vi "Main.vi"() -> ()   [LabVIEW 2026]
doc: "This template is for the Queued Message Handler design pattern.\n\nThe Event Handling Loop generates messages based on user interface actions.\n\nThe Message Handling Loop processes messages generated by the Event Handling Loop, or by other messages. The messages are string values, so new messages can be added easily to the Message Cases case structure in the Message Handling Loop. Each message cluster can also provide an optional value for Message Data, which is a variant that can be converted to whatever message-specific data is required."
uses:
  SubVIs/Controls/PCO_Config.ctl
  SubVIs/Controls/UI Data.ctl
  <instrlib>/PCO_SDK/File Group 0/vi.lib/Excelitas PCO GmbH/pco.labview/camera/Camera.lvclass
  SubVIs/Controls/TypeDef_FGV.ctl
  <instrlib>/PCO_SDK/File Group 0/vi.lib/Excelitas PCO GmbH/pco.labview/camera/Controls/binning.ctl
  SubVIs/QMH/Message Queue/Enqueue Message (Single).vi
  SubVIs/QMH/Message Queue/Message Queue.lvlib
  SubVIs/QMH/User Event - Stop/User Event - Stop.lvlib
panel:
  in  "Image Index":u32 max=9
  in  "Saving path":path
  in  "# of frames":u16=1 min=1 step=1
  out "FFT":T1(plugin-control)
  out "Camera":T1(plugin-control)
  in  "Stop live":bool
  in  "FFT?":bool
  in  "Grab":bool
  in  "Live":bool
  in  "PCO_Config":T2={"Exposure time (s)"=0.1, "TriggerMode"=0, "ROI X0"=1, "ROI Y0"=1, "ROI X1"=2048, "ROI Y1"=2048, "Binning"=1} {"TriggerMode" items=["auto sequence", "software trigger", "external exposure start", "external exposure control"]}
  out "Image dimensions (px)":dbl[](array[numeric])=[2048.0, 2048.0]
  out "Current task":string="\"Exit\" button pressed"
  in  "Exit":bool
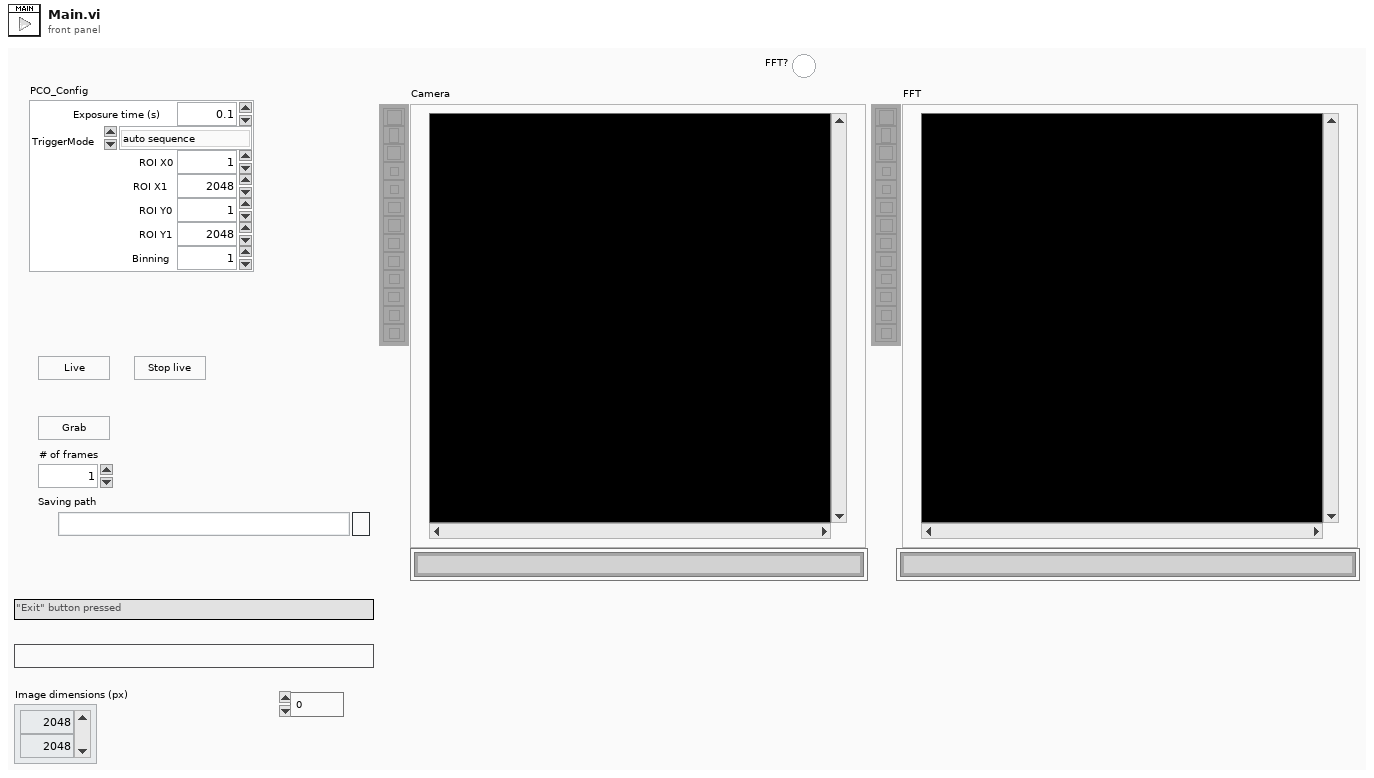
[diagram p1: front panel]
types:
  T1 = typedef "IMAQ Image.ctl" = refnum<image>
  T2 = typedef "PCO_Config.ctl" = cluster{"Exposure time (s)":dbl, "TriggerMode":u16, "ROI X0":u16, "ROI Y0":u16, "ROI X1":u16, "ROI Y1":u16, "Binning":u8}
  T3 = typedef "UI Data.ctl" = cluster{"Data Display Ref":refnum<vi>, "Exit Button Ref":refnum<vi>, "Message":string}
  T4 = typedef "Message Queue.lvlib/All Message Queues.ctl" = cluster{"UI":refnum<queue>, "Camera loop":refnum<queue>, "Display loop":refnum<queue>}
  T5 = typedef "TypeDef_FGV.ctl" = enum16{"Initialize", "Write", "Read"}
  T6 = typedef "Camera.lvclass/binning.ctl" = cluster{"vert":u16, "horz":u16, "mode":u16}
  T7 = cluster{"exposure_time_s":dbl, "delay_time_s":dbl, "roi":cluster{"x0":u64, "y0":u64, "x1":u64, "y1":u64}, "timestamp_mode":u16, "pixelrate":u32, "trigger_mode":u16, "acquire_mode":u16, "metadata_mode":u16, "noisefilter_mode":u16, "pixel_format":u32, "binning":T6, "auto_exposure":cluster{"region":u16, "min_exposure_s":dbl, "max_exposure_s":dbl}}
  T8 = enum16{"sequence", "sequence non blocking", "ring buffer", "fifo", "sequence_dpcore", "sequence_non_blocking_dpcore", "ring_buffer_dpcore", "fifo_dpcore", "tif", "multitif", "pcoraw", "b16", "dicom", "multidicom", "camram_ring", "camram_segment"}
  T9 = enum16{"Undefined", "Mono8", "Mono16", "BGRA8", "RGBA8", "BGRA16", "RGBA16", "CompressedMono8"}
  T10 = typedef "Image Type" = u32
  T11 = cluster{"serial":u32, "type":u16, "sub_type":u16, "interface_type":u16, "bit_resolution":u16, "min_exposure_time_s":dbl, "max_exposure_time_s":dbl, "min_exposure_step_s":dbl, "min_delay_time_s":dbl, "max_delay_time_s":dbl, "min_delay_step_s":dbl, "min_width":u64, "min_height":u64, "max_width":u64, "max_height":u64, "roi_step_horz":u64, "roi_step_vert":u64, "roi_symmetric_horz":bool, "roi_symmetric_vert":bool, "has_timestamp_mode":bool, "has_timestamp_mode_ascii_only":bool, "pixelrate_vec":u32[], "has_acquire_mode":bool, "has_ext_acquire_mode":bool, "has_metadata_mode":bool, "has_ram":bool, "binning_horz_vec":u16[], "binning_vert_vec":u16[], "has_average_binning":bool, "pixel_format_vec":u32[], "has_trigger_mode_extexpctrl":bool}
  T12 = cluster{"dwImgCounter":u32, "lvTimestamp":timestamp, "dwMicroSeconds":u32}[]
  T13 = cluster{"Plane 4 (alpha)":u16, "Plane 1 (Red)":u16, "Plane 2 (Green)":u16, "Plane 3 (Blue)":u16}[][][]
  T14 = cluster{"dwImgCounter":u32, "lvTimestamp":timestamp, "dwMicroSeconds":u32}
  T15 = typedef "IMAQ AVI2 Refnum.ctl" = refnum<k20>
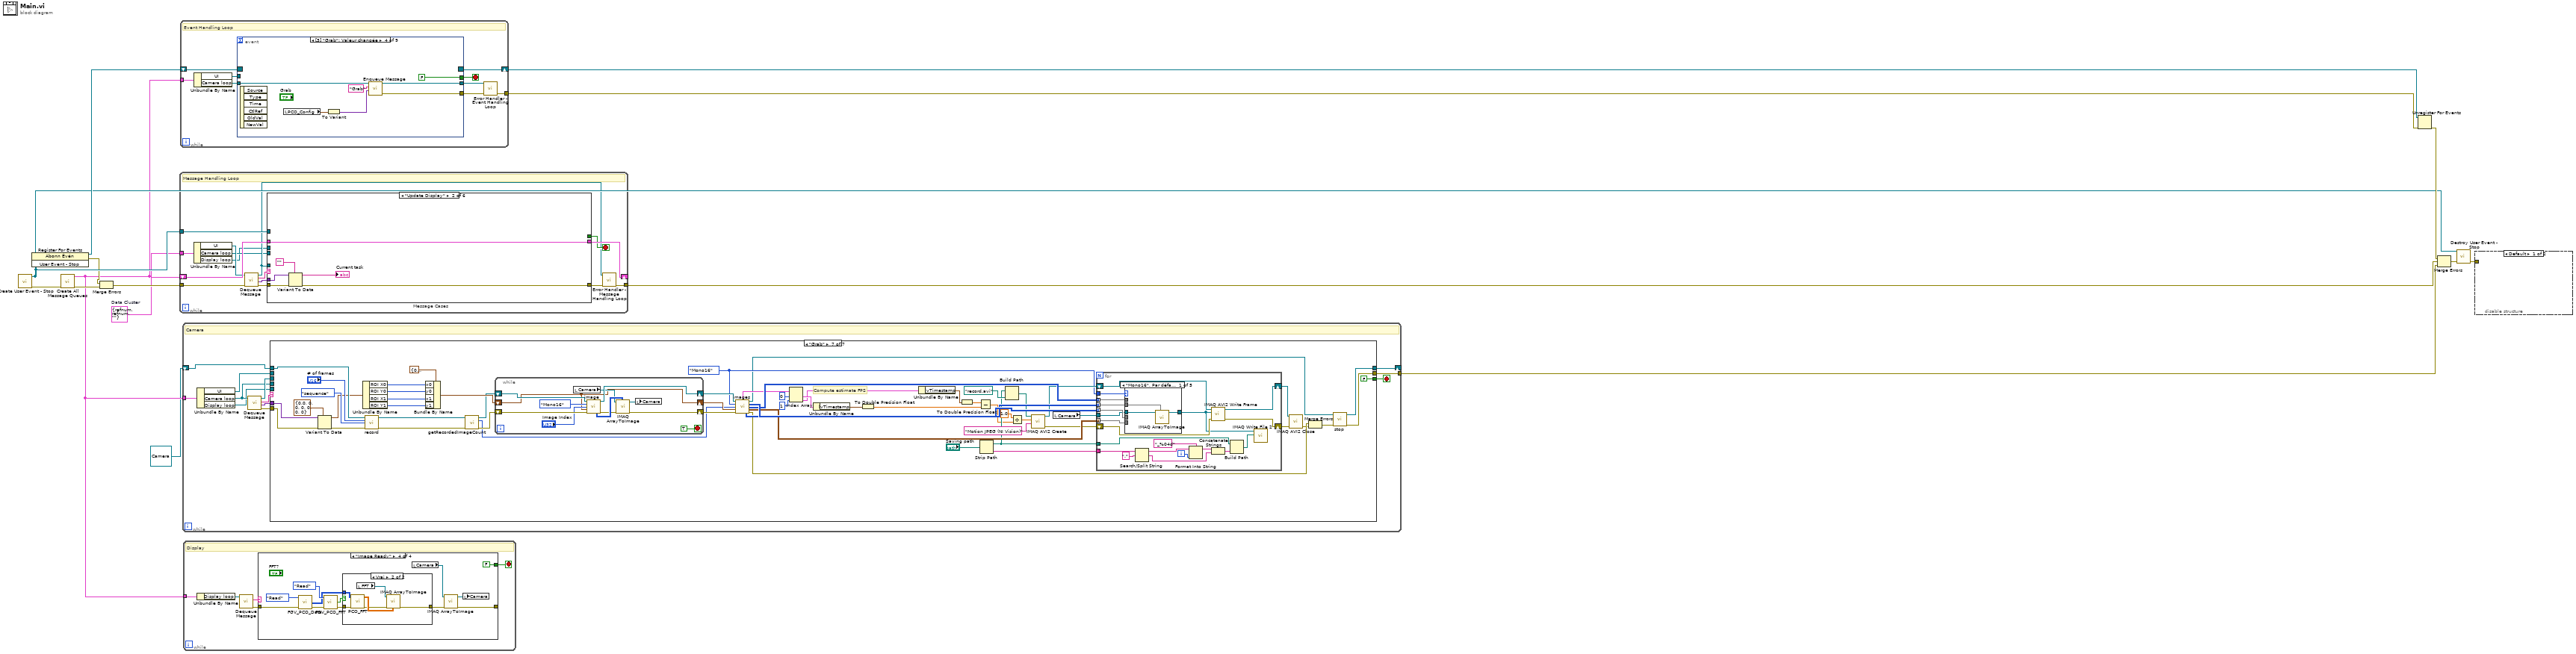
[diagram p0: block diagram]
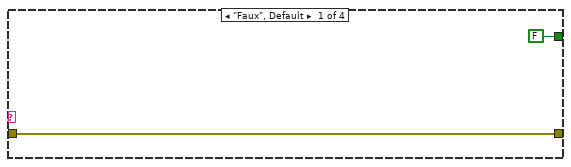
[diagram p2: hidden frame]
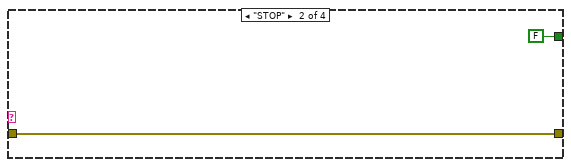
[diagram p3: hidden frame]
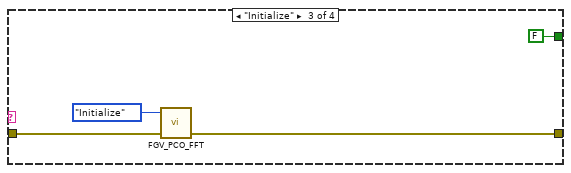
[diagram p4: hidden frame]
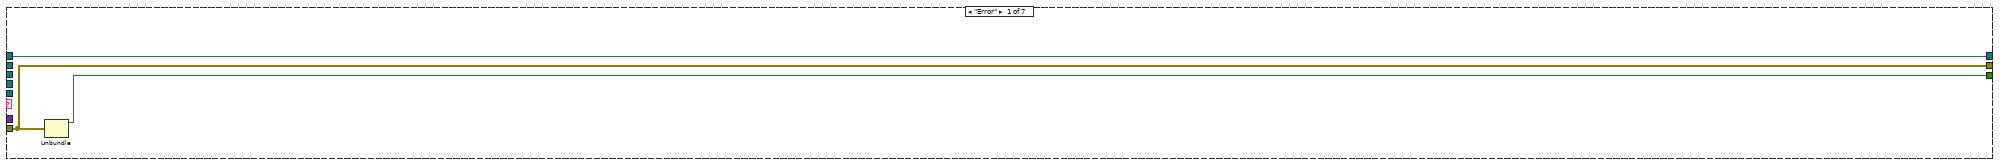
[diagram p6: hidden frame]
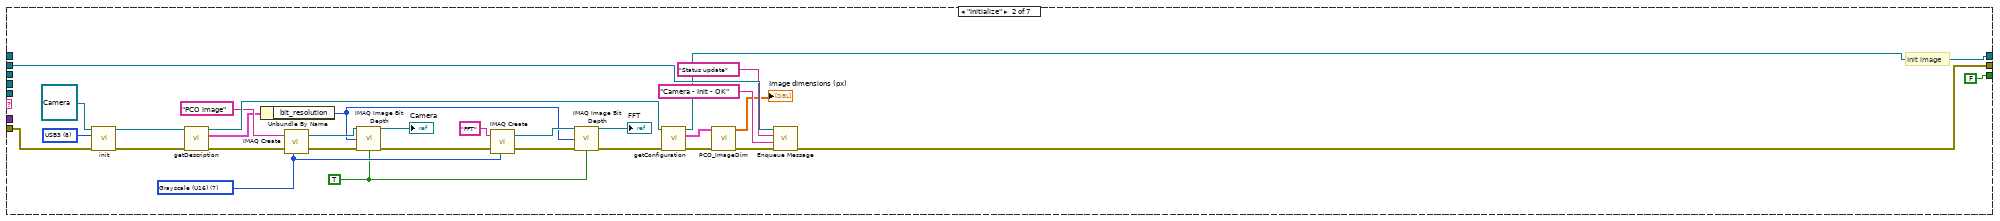
[diagram p7: hidden frame]
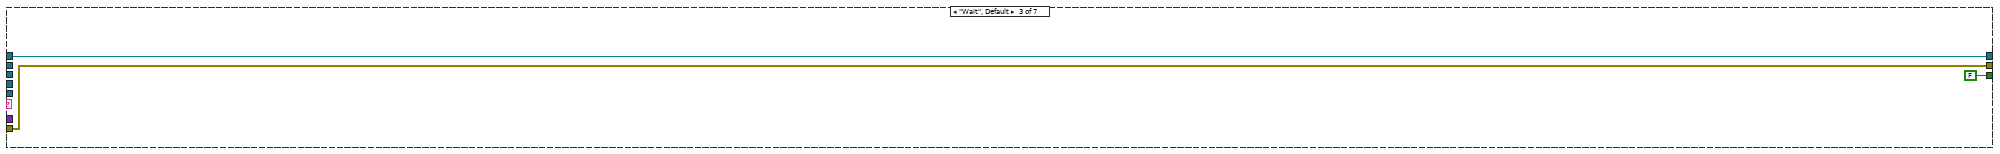
[diagram p8: hidden frame]
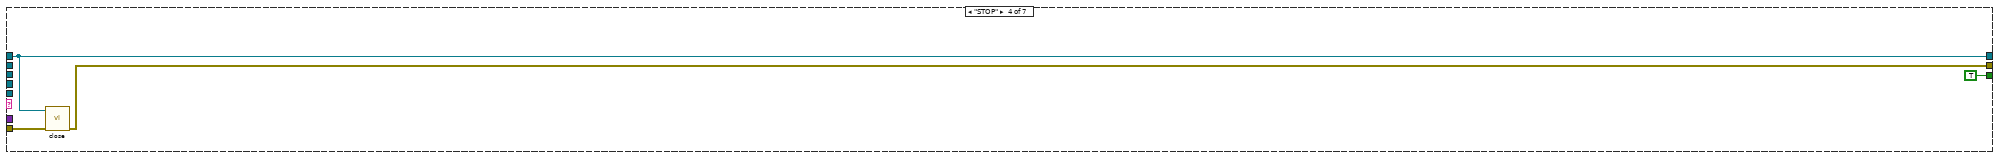
[diagram p9: hidden frame]
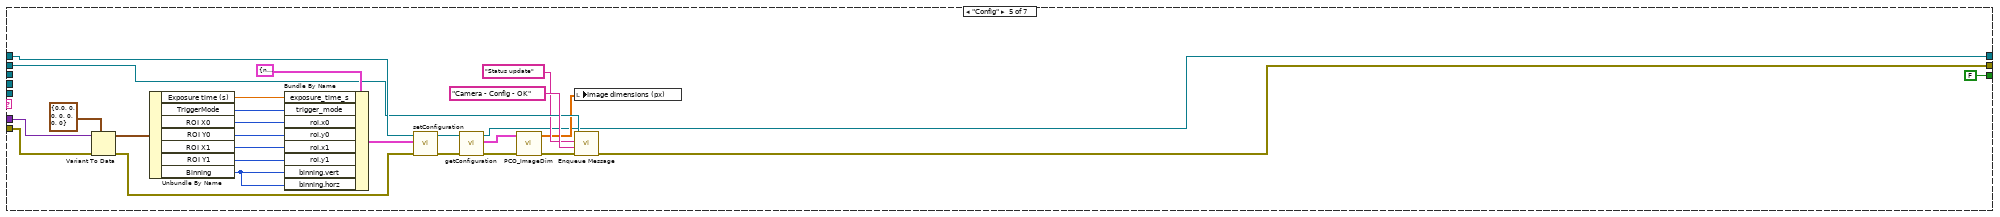
[diagram p10: hidden frame]
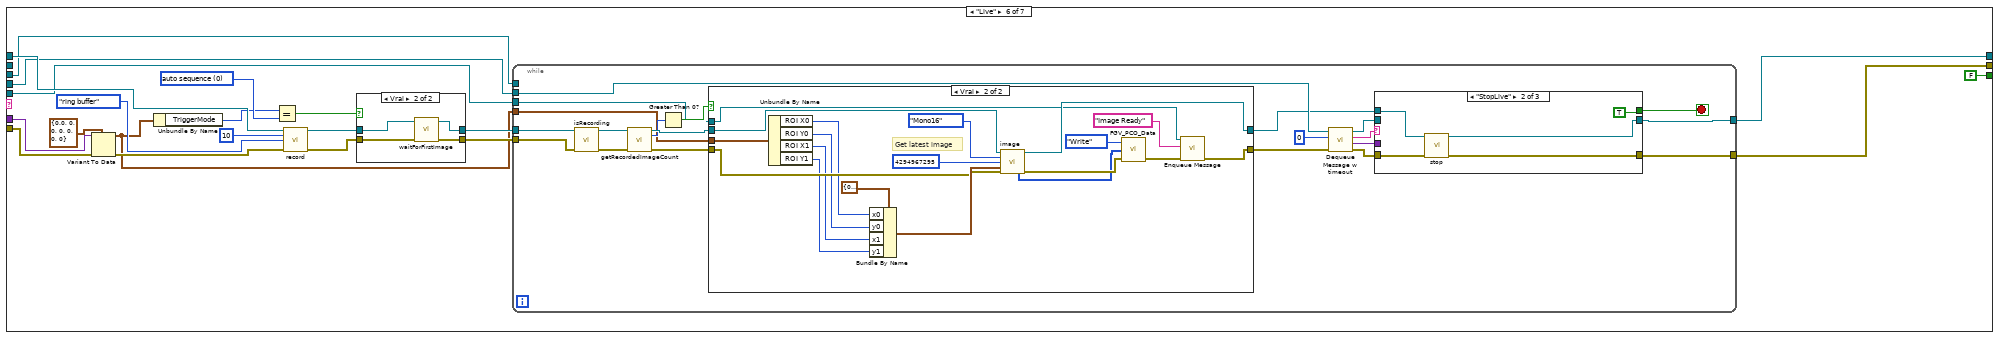
[diagram p11: hidden frame]
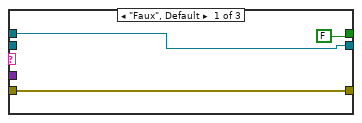
[diagram p12: hidden frame]
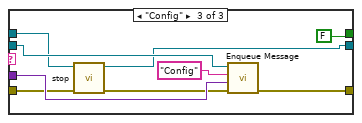
[diagram p13: hidden frame]
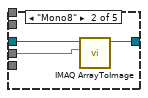
[diagram p16: hidden frame]
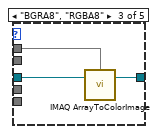
[diagram p17: hidden frame]
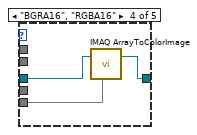
[diagram p18: hidden frame]
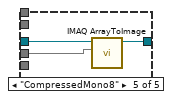
[diagram p19: hidden frame]
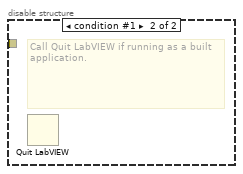
[diagram p20: hidden frame]
diagram:
  w4 = T3 {"Data Display Ref"=refnum, "Exit Button Ref"=refnum, "Message"=""}  # Data Cluster
  n1 = call "Create User Event - Stop.vi"() -> ("error out"=w14:errorcluster, "User Event - Stop"=w7:refnum<user-event>)  [unwired: 10 in]
  n2 = register-events(w7) -> (reference out=w8:refnum<event-registration>, error out=w5:errorcluster)  [unwired: 2 in]
  n3 = call "Create All Message Queues.vi"("error in (no error)"=w14) -> ("error out"=w16:errorcluster, "Message Queues out"=w2:T4)  [unwired: 9 in]
  n4 = Merge Errors(w5, w16) -> (w6:errorcluster)
  n5 = while {
    shift-right: [w30] -> _
    shift-left: w4 -> [w31]
    tunnel: w7 -> [w28]
    tunnel: w6 -> [w27]
    tunnel: [w22] -> w15
    tunnel: w2 -> [w20]
    stop <- w29 stop-if-true
    # "Message Handling Loop"
    n6 = Unbundle By Name(w20) -> ("UI"=w19:refnum<queue>, "Camera loop"=w18:refnum<queue>, "Display loop"=w17:refnum<queue>)
    n7 = call "Dequeue Message.vi"("error in (no error)"=w27, "Message Queue"=w19) -> ("error out"=w26:errorcluster, "Message Data"=w24:variant, "Message"=w25:string, "dup Message Queue"=w23:refnum<queue>)  [unwired: 6 in]
    n8 = case "Message Cases" shown="\"Update Display\"" w25 {
      tunnel: w23 -> [w34 _ _ w56 w70 _]
      tunnel: w26 -> [w39 w45 w52 w58 w71 w79]
      tunnel: [w40 w42 w47 w53 w66 w79] -> w21
      tunnel: w31 -> [w38 w46 w51 w57 w78 w80]
      tunnel: [w37 w46 w51 w57 w78 w80] -> w30
      tunnel: [_ _ _ _ TRUE _] -> w29
      tunnel: w24 -> [_ w44 w50 _ w74 _]
      tunnel: w28 -> [_ _ _ _ w76 _]
      tunnel: w18 -> [_ _ _ _ w69 _]
      tunnel: w17 -> [_ _ _ _ w59 _]
      frame "Initialize" {
        w32 = "Initial Message" ("Initial Message")
        n9 = control-ref of="Current task"() -> (w33:refnum<vi>)
        n10 = control-ref of="Exit"() -> (w36:refnum<vi>)
        n11 = Bundle By Name(cluster=w38, "Data Display Ref"=w33, "Exit Button Ref"=w36, "Message"=w32) -> (w37:T3)
        n12 = call-poly "Enqueue Message.vi"("error in (no error)"=w39, "Message Data"=w32, "Message"="Update Display", "Message Queue"=w34) -> ("error out"=w40:errorcluster)  [unwired: 6 in, 1 out]
      }
      frame "Update Display" {
        n13 = Variant To Data(error in=w45, type="", Variant=w44) -> (data=→"Current task":string, error out=w42:errorcluster)
      }
      frame "Error" {
        n14 = Variant To Data(error in=w52, type=errorcluster {"status"=FALSE, "code"=0, "source"=""} ("error constant"), Variant=w50) -> (data=w48:errorcluster, error out=w47:errorcluster)
        n15 = call <vilib>:"Simple Error Handler.vi"("error in (no error)"=w48) -> ()  [unwired: 4 in, 5 out]
      }
      frame "Confirm Quit" {
        n16 = call-poly "Enqueue Message.vi"("Priority Message? (F)"=TRUE, "error in (no error)"=w58, "Message"="Exit", "Message Queue"=w56) -> ("error out"=w53:errorcluster)  [unwired: 6 in, 1 out]
      }
      frame "Exit" {
        n17 = Variant To Data(error in=w71, type=errorcluster {"status"=FALSE, "code"=0, "source"=""} ("error constant"), Variant=w74) -> (error out=w67:errorcluster)  [unwired: 1 out]
        n18 = Release Queue(queue=w70, error in (no error)=w67) -> (error out=w65:errorcluster)  [unwired: 1 in, 2 out]
        n19 = call-poly "Enqueue Message.vi"("error in (no error)"=w65, "Message"="STOP", "Message Queue"=w69) -> ("error out"=w73:errorcluster, "dup Message Queue"=w72:refnum<queue>)  [unwired: 7 in]
        n20 = Release Queue(queue=w72, error in (no error)=w73) -> (error out=w61:errorcluster)  [unwired: 1 in, 2 out]
        n21 = call-poly "Enqueue Message.vi"("error in (no error)"=w61, "Message"="STOP", "Message Queue"=w59) -> ("error out"=w62:errorcluster, "dup Message Queue"=w63:refnum<queue>)  [unwired: 7 in]
        n22 = Release Queue(queue=w63, error in (no error)=w62) -> (error out=w60:errorcluster)  [unwired: 1 in, 2 out]
        n23 = call "Fire User Event - Stop.vi"("error in (no error)"=w60, "User Event - Stop"=w76) -> ("error out"=w66:errorcluster)  [unwired: 9 in]
      }
      frame Default {
      }
    }
    n24 = call "Error Handler - Message Handling Loop.vi"("error in (no error)"=w21, "Message Queue"=w23) -> ("dup error in"=w22:errorcluster)  [unwired: 8 in, 1 out]
  }
  n25 = while {
    shift-right: [w88] -> w11
    shift-left: w8 -> [w89]
    tunnel: [w84] -> w9
    tunnel: w2 -> [w81]
    stop <- w86 stop-if-true
    # "Event Handling Loop"
    n26 = Unbundle By Name(w81) -> ("UI"=w83:refnum<queue>, "Camera loop"=w82:refnum<queue>)
    n27 = event shown="[3] \"Grab\": Valeur changée" {
      selector: w89 -> [_ _ _ _ _ _ _ _ _]
      dyn-events: [_ _ _ _ _ _ _ _ _] -> w88
      timeout: _ -> [_ _ _ _ _ _ _ _ _]
      tunnel: [FALSE ("Discard?") FALSE ("Discard?") _ FALSE ("Discard?") FALSE ("Discard?") FALSE ("Discard?") FALSE ("Discard?") FALSE ("Discard?") TRUE ("Discard?")] -> w86
      tunnel: w83 -> [w95 w105 _ _ w123 _ w131 w138 w142]
      tunnel: [w94 w101 w108 w115 w121 w126 errorcluster {"status"=FALSE, "code"=0, "source"=""} ("error out") w132 errorcluster {"status"=FALSE, "code"=0, "source"=""} ("error out")] -> w87
      tunnel: [w93 w105 w107 w116 w123 w125 w131 w137 w142] -> w85
      tunnel: w82 -> [_ w99 w106 w117 _ w127 _ _ _]
      event Panel Close? {
        n28 = event-data() -> ()  [unwired: 1 in, 1 out]
        n29 = call-poly "Enqueue Message.vi"("Priority Message? (F)"=TRUE, "Message"="Confirm Quit", "Message Queue"=w95) -> ("error out"=w94:errorcluster, "dup Message Queue"=w93:refnum<queue>)  [unwired: 7 in]
        n30 = event-data("Discard?"=TRUE) -> ()  [unwired: 1 in, 1 out]
      }
      event Value Change {
        n31 = event-data() -> ()  [unwired: 1 in, 6 out]
        n32 = To Variant(anything="PCO_Config") -> (Variant=w102:variant)
        n33 = Flush Queue(queue=w99) -> (queue out=w97:refnum<queue>, error out=w98:errorcluster)  [unwired: 1 in, 1 out]
        n34 = call-poly "Enqueue Message.vi"("error in (no error)"=w98, "Message Data"=w102, "Message"="Config", "Message Queue"=w97) -> ("error out"=w101:errorcluster)  [unwired: 6 in, 1 out]
      }
      event "Live": Value Change {
        n35 = event-data() -> ()  [unwired: 1 in, 6 out]
        n36 = local read "PCO_Config"() -> (w111:T2)
        n37 = To Variant(anything=w111) -> (Variant=w110:variant)
        n38 = call-poly "Enqueue Message.vi"("Message Data"=w110, "Message"="Live", "Message Queue"=w106) -> ("error out"=w108:errorcluster, "dup Message Queue"=w107:refnum<queue>)  [unwired: 7 in]
      }
      event "Grab": Value Change {
        n39 = event-data() -> ()  [unwired: 1 in, 6 out]
        n40 = local read "PCO_Config"() -> (w113:T2)
        n41 = To Variant(anything=w113) -> (Variant=w112:variant)
        n42 = call-poly "Enqueue Message.vi"("Message Data"=w112, "Message"="Grab", "Message Queue"=w117) -> ("error out"=w115:errorcluster, "dup Message Queue"=w116:refnum<queue>)  [unwired: 7 in]
      }
      event "FFT?": Value Change {
        n43 = event-data() -> ("NewVal"=w119:bool)  [unwired: 1 in]
        n44 = call "FGV_PCO_FFT.vi"("FFT?"=w119, "Action"=TypeDef_FGV."Write") -> ("error out"=w121:errorcluster)  [unwired: 2 in, 1 out]
      }
      event "Stop live": Value Change {
        n45 = event-data() -> ()  [unwired: 1 in, 6 out]
        n46 = call-poly "Enqueue Message.vi"("Message"="StopLive", "Message Queue"=w127) -> ("error out"=w126:errorcluster, "dup Message Queue"=w125:refnum<queue>)  [unwired: 8 in]
      }
      event Application Instance Close {
        n47 = event-data() -> ()  [unwired: 1 in, 1 out]
      }
      event "Exit": Value Change {
        n48 = event-data() -> ()  [unwired: 1 in, 1 out]
        n49 = call-poly "Enqueue Message.vi"("Priority Message? (F)"=TRUE, "Message Data"=errorcluster {"status"=FALSE, "code"=0, "source"=""} ("error constant"), "Message"="Exit", "Message Queue"=w138) -> ("error out"=w132:errorcluster, "dup Message Queue"=w137:refnum<queue>)  [unwired: 6 in]
      }
      event User Event {
        n50 = event-data() -> ()  [unwired: 1 in, 1 out]
        n51 = local write "Current task"("\"Exit\" button pressed" ("VI Stopped")) -> ()
      }
    }
    n52 = call "Error Handler - Event Handling Loop.vi"("error in (no error)"=w87, "Message Queue"=w85) -> ("dup error in"=w84:errorcluster)  [unwired: 8 in, 1 out]
  }
  n53 = while {
    tunnel: [w150] -> w3
    tunnel: w2 -> [w148]
    shift-right: [w146] -> _
    shift-left: refnum<class "Camera.lvclass"> refnum ("Camera out") -> [w145]
    stop <- w151 stop-if-true
    # "Camera"
    n54 = Unbundle By Name(w148) -> ("UI"=w147:refnum<queue>, "Camera loop"=w144:refnum<queue>, "Display loop"=w143:refnum<queue>)
    n55 = call "Dequeue Message.vi"("Message Queue"=w144) -> ("error out"=w154:errorcluster, "Message Data"=w152:variant, "Message"=w153:string, "dup Message Queue"=w149:refnum<queue>)  [unwired: 7 in]
    n56 = case shown="\"Grab\"" w153 {
      tunnel: w154 -> [w157 w181 w191 w194 w221 w238 w357]
      tunnel: w152 -> [_ _ _ _ w220 w234 w356]
      tunnel: w147 -> [_ w188 _ _ w205 _ _]
      tunnel: [w156 FALSE ("status") FALSE ("status") TRUE FALSE ("status") FALSE ("status") FALSE ("status")] -> w151
      tunnel: [w157 w173 w191 w193 w204 w226 w311] -> w150
      tunnel: w149 -> [_ _ _ _ _ w229 _]
      tunnel: [w155 w178 w190 w192 w196 w225 w309] -> w146
      tunnel: w145 -> [w155 _ w190 w192 w215 w242 w363]
      tunnel: w144 -> [_ _ _ _ _ w228 _]
      tunnel: w143 -> [_ _ _ _ _ w227 _]
      frame "Error" {
        n57 = Unbundle(w157) -> ("status"=w156:bool)  [unwired: 2 out]
      }
      frame "Initialize" {
        w159 = TRUE ("Get/Set Bit Depth? (Set)")
        w164 = T10 7 items=["Grayscale (U8)", "Grayscale (I16)", "Grayscale (SGL)", "Complex (CSG)", "RGB (U32)", "HSL (U32)", "RGB (U64)", "Grayscale (U16)"] ("Image Type")
        w180 = u16 8 items=["FireWire"=1, "GenICam"=3, "GigE"=5, "USB"=6, "CameraLinkME4"=7, "USB3"=8, "CLHS"=11, "All"=65535] ("interface")
        # "Init image"
        n58 = call-dynamic "init.vi"("Camera in"=refnum<class "Camera.lvclass"> refnum, "interface"=w180, "error in (no error)"=w181) -> ("Camera out"=w184:refnum<class "Camera.lvclass">, "error out"=w183:errorcluster)  [unwired: 6 in]
        n59 = call-dynamic "getDescription.vi"("error in (no error)"=w183, "Camera in"=w184) -> ("error out"=w167:errorcluster, "description"=w170:T11, "Camera out"=w179:refnum<class "Camera.lvclass">)  [unwired: 7 in]
        n60 = Unbundle By Name(w170) -> ("bit_resolution"=w160:u16)
        n61 = call "IMAQ Create"("Image Name"="PCO Image", "Image Type"=w164, "error in (no error)"=w167) -> ("New Image"=w169:T1, "error out"=w168:errorcluster)  [unwired: 2 in]
        n62 = call "IMAQ Image Bit Depth"("Image"=w169, "Bit Depth (0)"=w160, "error in (no error)"=w168, "Get/Set Bit Depth? (Set)"=w159) -> ("Image Out"=→"Camera":T1, "error out"=w165:errorcluster)  [unwired: 9 in, 1 out]
        n63 = call "IMAQ Create"("Image Name"="FFT", "Image Type"=w164, "error in (no error)"=w165) -> ("New Image"=w162:T1, "error out"=w163:errorcluster)  [unwired: 2 in]
        n64 = call "IMAQ Image Bit Depth"("Image"=w162, "Bit Depth (0)"=w160, "error in (no error)"=w163, "Get/Set Bit Depth? (Set)"=w159) -> ("Image Out"=→"FFT":T1, "error out"=w158:errorcluster)  [unwired: 9 in, 1 out]
        n65 = call-dynamic "getConfiguration.vi"("error in (no error)"=w158, "Camera in"=w179) -> ("error out"=w176:errorcluster, "configuration"=w177:T7, "Camera out"=w178:refnum<class "Camera.lvclass">)  [unwired: 7 in]
        n66 = call "PCO_ImageDim.vi"("error in"=w176, "configuration"=w177) -> ("error out"=w175:errorcluster, "Dimensions"=→"Image dimensions (px)":dbl[])  [unwired: 8 in]
        n67 = call-poly "Enqueue Message.vi"("error in (no error)"=w175, "Message Data"="Camera - Init - OK", "Message"="Status update", "Message Queue"=w188) -> ("error out"=w173:errorcluster)  [unwired: 6 in, 1 out]
      }
      frame "Wait", Default {
      }
      frame "STOP" {
        n68 = call-dynamic "close.vi"("error in (no error)"=w194, "Camera in"=w192) -> ("error out"=w193:errorcluster)  [unwired: 9 in]
      }
      frame "Config" {
        n69 = Variant To Data(error in=w221, type=T2 {"Exposure time (s)"=0.0, "TriggerMode"=0, "ROI X0"=0, "ROI Y0"=0, "ROI X1"=0, "ROI Y1"=0, "Binning"=0} ("PCO_Config"), Variant=w220) -> (data=w217:T2, error out=w216:errorcluster)
        n70 = Unbundle By Name(w217) -> ("Exposure time (s)"=w213:dbl, "TriggerMode"=w212:u16, "ROI X0"=w207:u16, "ROI Y0"=w208:u16, "ROI X1"=w209:u16, "ROI Y1"=w210:u16, "Binning"=w211:u8)
        n71 = Bundle By Name(cluster=T7 {"exposure_time_s"=nan, "delay_time_s"=nan, "roi"={"x0"=18446744073709551615, "y0"=18446744073709551615, "x1"=18446744073709551615, "y1"=18446744073709551615}, "timestamp_mode"=65535, "pixelrate"=4294967295, "trigger_mode"=65535, "acquire_mode"=65535, "metadata_mode"=65535, "noisefilter_mode"=65535, "pixel_format"=4294967295, "binning"={"vert"=65535, "horz"=65535, "mode"=0}, "auto_exposure"={"region"=0, "min_exposure_s"=0.001, "max_exposure_s"=0.1}} ("configuration"), "exposure_time_s"=w213, "trigger_mode"=w212, "roi.x0"=w207, "roi.y0"=w208, "roi.x1"=w209, "roi.y1"=w210, "binning.vert"=w211, "binning.horz"=w211) -> (w214:T7)
        n72 = call-dynamic "setConfiguration.vi"("error in (no error)"=w216, "configuration"=w214, "Camera in"=w215) -> ("error out"=w198:errorcluster, "Camera out"=w199:refnum<class "Camera.lvclass">)  [unwired: 7 in]
        n73 = call-dynamic "getConfiguration.vi"("error in (no error)"=w198, "Camera in"=w199) -> ("error out"=w202:errorcluster, "configuration"=w201:T7, "Camera out"=w196:refnum<class "Camera.lvclass">)  [unwired: 7 in]
        n74 = call "PCO_ImageDim.vi"("error in"=w202, "configuration"=w201) -> ("error out"=w197:errorcluster, "Dimensions"=w200:dbl[])  [unwired: 8 in]
        n75 = local write "Image dimensions (px)"(w200) -> ()
        n76 = call-poly "Enqueue Message.vi"("error in (no error)"=w197, "Message Data"="Camera - Config - OK", "Message"="Status update", "Message Queue"=w205) -> ("error out"=w204:errorcluster)  [unwired: 6 in, 1 out]
      }
      frame "Live" {
        w236 = u16 0 items=["auto sequence", "software trigger", "external exposure start", "external exposure control"] ("TriggerMode")
        n77 = Variant To Data(error in=w238, type=T2 {"Exposure time (s)"=0.0, "TriggerMode"=0, "ROI X0"=0, "ROI Y0"=0, "ROI X1"=0, "ROI Y1"=0, "Binning"=0} ("PCO_Config"), Variant=w234) -> (data=w230:T2, error out=w237:errorcluster)
        n78 = Unbundle By Name(w230) -> ("TriggerMode"=w235:u16)
        n79 = Equal?(x=w235, y=w236) -> (x = y?=w233:bool)
        n80 = call-dynamic "record.vi"("Camera in"=w242, "num_images"=u32 10 ("dwImgCount"), "record_mode"=T8."ring buffer", "error in (no error)"=w237) -> ("Camera out"=w223:refnum<class "Camera.lvclass">, "error out"=w224:errorcluster)  [unwired: 10 in]
        n81 = case shown="Vrai" w233 {
          tunnel: w224 -> [w303 w308]
          tunnel: w223 -> [w304 w307]
          tunnel: [w304 w306] -> w231
          tunnel: [w303 w305] -> w232
          frame False {
          }
          frame True {
            n82 = call-dynamic "waitForFirstImage.vi"("error in (no error)"=w308, "Camera in"=w307) -> ("error out"=w305:errorcluster, "Camera out"=w306:refnum<class "Camera.lvclass">)  [unwired: 8 in]
          }
        }
        n83 = while {
          tunnel: w232 -> [w258]
          tunnel: w231 -> [w257]
          tunnel: w230 -> [w256]
          tunnel: w229 -> [_]
          tunnel: w228 -> [w254]
          tunnel: w227 -> [w252]
          tunnel: [w247] -> w226
          tunnel: [w246] -> w225
          stop <- w245 stop-if-true
          n84 = call-dynamic "isRecording.vi"("Camera in"=w257, "error in (no error)"=w258) -> ("Camera out"=w264:refnum<class "Camera.lvclass">, "error out"=w263:errorcluster)  [unwired: 11 in, 1 out]
          n85 = call-dynamic "getRecordedImageCount.vi"("Camera in"=w264, "error in (no error)"=w263) -> ("Camera out"=w261:refnum<class "Camera.lvclass">, "recorded_image_count"=w259:u32, "error out"=w262:errorcluster)  [unwired: 11 in]
          n86 = Greater Than 0?(x=w259) -> (x > 0?=w260:bool)
          n87 = case shown="Vrai" w260 {
            tunnel: [w282 w288] -> w255
            tunnel: w262 -> [w282 w299]
            tunnel: w261 -> [w283 w298]
            tunnel: [w283 w297] -> w248
            tunnel: w256 -> [_ w296]
            tunnel: w252 -> [_ w290]
            frame False {
            }
            frame True {
              # "Get latest image"
              n88 = Unbundle By Name(w296) -> ("ROI X0"=w295:u16, "ROI Y0"=w294:u16, "ROI X1"=w293:u16, "ROI Y1"=w292:u16)
              n89 = Bundle By Name(cluster=cluster{"x0":u64, "y0":u64, "x1":u64, "y1":u64} {"x0"=0, "y0"=0, "x1"=0, "y1"=0} ("roi"), "x0"=w295, "y0"=w294, "x1"=w293, "y1"=w292) -> (w300:cluster{"x0":u64, "y0":u64, "x1":u64, "y1":u64})
              n90 = call-dynamic "image.vi"("Camera in"=w298, "data_format"=T9."Mono16", "image_index"=u32 4294967295 ("dwImgIdx"), "roi"=w300, "error in (no error)"=w299) -> ("Camera out"=w297:refnum<class "Camera.lvclass">, "raw_image (U16)"=w284:u16[][], "error out"=w286:errorcluster)  [unwired: 2 in, 6 out]
              n91 = call "FGV_PCO_Data.vi"("error in"=w286, "Data"=w284, "Action"=TypeDef_FGV."Write") -> ("error out"=w285:errorcluster)  [unwired: 1 in, 1 out]
              n92 = call-poly "Enqueue Message.vi"("error in (no error)"=w285, "Message"="Image Ready", "Message Queue"=w290) -> ("error out"=w288:errorcluster)  [unwired: 7 in, 1 out]
            }
          }
          n93 = call "Dequeue Message w timeout.vi"("entrée d'erreur (pas d'erreur)"=w255, "timeout en ms (-1)"=0, "Message Queue"=w254) -> ("sortie d'erreur"=w250:errorcluster, "Message Data"=w249:variant, "Message"=w253:string, "Message Queue"=w251:refnum<queue>)  [unwired: 5 in]
          n94 = case shown="\"StopLive\"" w253 {
            tunnel: w251 -> [_ _ w281]
            tunnel: w250 -> [w266 w271 w276]
            tunnel: w249 -> [_ _ w279]
            tunnel: w248 -> [w267 w272 w277]
            tunnel: [w266 w270 w274] -> w247
            tunnel: [w267 w269 w278] -> w246
            tunnel: [FALSE TRUE FALSE] -> w245
            frame "Faux", Default {
            }
            frame "StopLive" {
              n95 = call-dynamic "stop.vi"("error in (no error)"=w271, "Camera in"=w272) -> ("error out"=w270:errorcluster, "Camera out"=w269:refnum<class "Camera.lvclass">)  [unwired: 8 in]
            }
            frame "Config" {
              n96 = call-dynamic "stop.vi"("error in (no error)"=w276, "Camera in"=w277) -> ("error out"=w275:errorcluster, "Camera out"=w278:refnum<class "Camera.lvclass">)  [unwired: 8 in]
              n97 = call-poly "Enqueue Message.vi"("error in (no error)"=w275, "Message Data"=w279, "Message"="Config", "Message Queue"=w281) -> ("error out"=w274:errorcluster)  [unwired: 6 in, 1 out]
            }
          }
        }
      }
      frame "Grab" {
        w315 = T9."Mono16" ("data_format")
        # "Compute estimate FPS"
        n98 = Variant To Data(error in=w357, type=T2 {"Exposure time (s)"=0.0, "TriggerMode"=0, "ROI X0"=0, "ROI Y0"=0, "ROI X1"=0, "ROI Y1"=0, "Binning"=0} ("PCO_Config"), Variant=w356) -> (data=w354:T2, error out=w355:errorcluster)
        n99 = Unbundle By Name(w354) -> ("ROI X0"=w353:u16, "ROI Y0"=w352:u16, "ROI X1"=w351:u16, "ROI Y1"=w350:u16)
        n100 = call-dynamic "record.vi"("Camera in"=w363, "num_images"="# of frames", "record_mode"=T8."sequence", "error in (no error)"=w355) -> ("Camera out"=w362:refnum<class "Camera.lvclass">, "error out"=w361:errorcluster)  [unwired: 10 in]
        n101 = Bundle By Name(cluster=cluster{"x0":u64, "y0":u64, "x1":u64, "y1":u64} {"x0"=0, "y0"=0, "x1"=0, "y1"=0} ("roi"), "x0"=w353, "y0"=w352, "x1"=w351, "y1"=w350) -> (w359:cluster{"x0":u64, "y0":u64, "x1":u64, "y1":u64})
        n102 = call-dynamic "getRecordedImageCount.vi"("Camera in"=w362, "error in (no error)"=w361) -> ("Camera out"=w348:refnum<class "Camera.lvclass">, "recorded_image_count"=w316:u32, "error out"=w349:errorcluster)  [unwired: 11 in]
        n103 = while {
          shift-right: [w411] -> w346
          shift-left: w348 -> [w413]
          shift-right: [w404] -> w347
          shift-left: w349 -> [w412]
          shift-right: [w403] -> w317
          shift-left: w359 -> [w403]
          stop <- TRUE stop-if-true
          n104 = local read "Camera"() -> (w408:T1)
          n105 = call-dynamic "image.vi"("Camera in"=w413, "data_format"=T9."Mono16", "image_index"="Image Index", "roi"=w403, "error in (no error)"=w412) -> ("Camera out"=w411:refnum<class "Camera.lvclass">, "raw_image (U16)"=w409:u16[][], "error out"=w405:errorcluster)  [unwired: 2 in, 6 out]
          n106 = call "IMAQ ArrayToImage"("Image Pixels (U16)"=w409, "error in (no error)"=w405, "Image"=w408) -> ("error out"=w404:errorcluster, "Image Out"=w407:T1)  [unwired: 7 in]
          n107 = local write "Camera"(w407) -> ()
        }
        n108 = call-dynamic "images.vi"("Camera in"=w346, "data_format"=w315, "image_count"=w316, "roi"=w317, "error in (no error)"=w347) -> ("timestamp_list"=w330:T12, "Camera out"=w310:refnum<class "Camera.lvclass">, "image_list (U8)"=w345:u8[][][], "image_list (U32)"=w343:u32[][][], "image_list (U64)"=w342:T13, "raw_image_list (U16)"=w344:u16[][][], "error out"=w337:errorcluster)  [unwired: 2 in, 2 out]
        n109 = Index Array(array=w330, index #1=0 ("index"), index #2=1 ("index")) -> (element #1=w327:T14, element #2=w326:T14)
        n110 = Unbundle By Name(w327) -> ("lvTimestamp"=w325:timestamp)
        n111 = To Double Precision Float(number=w325) -> (double precision float=w322:dbl)
        n112 = Unbundle By Name(w326) -> ("lvTimestamp"=w324:timestamp)
        n113 = To Double Precision Float(number=w324) -> (double precision float=w323:dbl)
        n114 = Subtract(x=w323, y=w322) -> (x-y=w321:dbl)
        n115 = Strip Path(path="Saving path") -> (stripped path=w331:path, name=w334:string)
        n116 = Build Path(base path=w331, name or relative path=path "record.avi") -> (appended path=w332:path)
        n117 = Divide(x=1.0, y=w321) -> (x/y=w319:dbl)
        n118 = call "IMAQ AVI2 Create"("Codec"="Motion JPEG (NI Vision)", "Frames Per Second"=w319, "AVI Path"=w332) -> ("error out"=w341:errorcluster, "AVI Refnum"=w340:T15)  [unwired: 7 in]
        n119 = local read "Camera"() -> (w335:T1)
        n120 = for {
          tunnel: w345 -> [w386] mode=indexing
          tunnel: w344 -> [w385] mode=indexing
          tunnel: w343 -> [w384] mode=indexing
          tunnel: w342 -> [w383] mode=indexing
          shift-right: [w379] -> w338
          shift-left: w340 -> [w382]
          shift-right: [w380] -> w339
          shift-left: w341 -> [w381]
          tunnel: w335 -> [w369]
          tunnel: w315 -> [w368]
          tunnel: w334 -> [w367]
          tunnel: w331 -> [w366]
          i -> [w371]
          n121 = case shown="\"Mono16\", Par défaut" w368 {
            tunnel: w369 -> [w389 w392 w395 w398 w401]
            tunnel: [w387 w390 w394 w396 w400] -> w378
            tunnel: w383 -> [_ _ _ w397 _]
            tunnel: w384 -> [_ _ w393 _ _]
            tunnel: w386 -> [_ w391 _ _ w399]
            tunnel: w385 -> [w388 _ _ _ _]
            frame "Mono16", Default {
              n122 = call "IMAQ ArrayToImage"("Image Pixels (U16)"=w388, "Image"=w389) -> ("Image Out"=w387:T1)  [unwired: 8 in, 1 out]
            }
            frame "Mono8" {
              n123 = call "IMAQ ArrayToImage"("Image Pixels (U8)"=w391, "Image"=w392) -> ("Image Out"=w390:T1)  [unwired: 8 in, 1 out]
            }
            frame "BGRA8", "RGBA8" {
              n124 = call "IMAQ ArrayToColorImage"("Image Pixels (U32)"=w393, "Image"=w395) -> ("Image Out"=w394:T1)  [unwired: 3 in, 1 out]
            }
            frame "BGRA16", "RGBA16" {
              n125 = call "IMAQ ArrayToColorImage"("Image"=w398, "Image Pixels (U64)"=w397) -> ("Image Out"=w396:T1)  [unwired: 3 in, 1 out]
            }
            frame "CompressedMono8" {
              n126 = call "IMAQ ArrayToImage"("Image Pixels (U8)"=w399, "Image"=w401) -> ("Image Out"=w400:T1)  [unwired: 8 in, 1 out]
            }
          }
          n127 = Search/Split String(string=w367, search string/char (-)=".") -> (substring before match=w375:string, match + rest of string=w376:string)  [unwired: 1 in, 1 out]
          n128 = Format Into String(format string="_%04d", initial string=w375, w371) -> (resulting string=w377:string)  [unwired: 1 in, 1 out]
          n129 = call "IMAQ AVI2 Write Frame"("error in (no error)"=w381, "Image"=w378, "AVI Refnum"=w382) -> ("error out"=w380:errorcluster, "AVI Refnum (duplicate)"=w379:T15)  [unwired: 6 in, 1 out]
          n130 = Concatenate Strings(w377, w376) -> (w372:string)
          n131 = Build Path(base path=w366, name or relative path=w372) -> (appended path=w370:path)
          n132 = call-poly "IMAQ Write File 2"("File Path"=w370, "Image"=w378) -> ()  [unwired: 8 in, 2 out]
        }
        n133 = call "IMAQ AVI2 Close"("error in (no error)"=w339, "AVI Refnum"=w338) -> ("error out"=w336:errorcluster)  [unwired: 9 in]
        n134 = Merge Errors(w337, w336) -> (w312:errorcluster)
        n135 = call-dynamic "stop.vi"("error in (no error)"=w312, "Camera in"=w310) -> ("error out"=w311:errorcluster, "Camera out"=w309:refnum<class "Camera.lvclass">)  [unwired: 8 in]
      }
    }
  }
  n136 = while {
    tunnel: w2 -> [w418]
    stop <- w414 stop-if-true
    # "Display"
    n137 = Unbundle By Name(w418) -> ("Display loop"=w417:refnum<queue>)
    n138 = call "Dequeue Message.vi"("Message Queue"=w417) -> ("error out"=w415:errorcluster, "Message"=w416:string)  [unwired: 7 in, 2 out]
    n139 = case shown="\"Image Ready\"" w416 {
      tunnel: w415 -> [w420 w421 w425 w435]
      tunnel: [w420 w421 w424 w434] -> _
      tunnel: [FALSE FALSE FALSE FALSE] -> w414
      frame "Faux", Default {
      }
      frame "STOP" {
      }
      frame "Initialize" {
        n140 = call "FGV_PCO_FFT.vi"("error in"=w425, "Action"=TypeDef_FGV."Initialize") -> ("error out"=w424:errorcluster)  [unwired: 2 in, 1 out]
      }
      frame "Image Ready" {
        n141 = call "FGV_PCO_Data.vi"("error in"=w435, "Action"=TypeDef_FGV."Read") -> ("error out"=w431:errorcluster, "Data"=w427:u16[][])  [unwired: 2 in]
        n142 = call "FGV_PCO_FFT.vi"("error in"=w431, "Action"=TypeDef_FGV."Read") -> ("error out"=w429:errorcluster, "FFT?"=w428:bool)  [unwired: 2 in]
        n143 = case shown="Vrai" w428 {
          tunnel: [w439 w440] -> w430
          tunnel: w429 -> [w439 w444]
          tunnel: w427 -> [_ w443]
          frame False {
          }
          frame True {
            n144 = call "PCO_FFT.vi"("error in (no error)"=w444, "Data"=w443) -> ("error out"=w441:errorcluster, "FFT"=w442:dbl[][])  [unwired: 8 in]
            n145 = local read "FFT"() -> (w445:T1)
            n146 = call "IMAQ ArrayToImage"("Image Pixels (Float)"=w442, "error in (no error)"=w441, "Image"=w445) -> ("error out"=w440:errorcluster)  [unwired: 7 in, 1 out]
          }
        }
        n147 = local read "Camera"() -> (w437:T1)
        n148 = call "IMAQ ArrayToImage"("error in (no error)"=w430, "Image"=w437) -> ("error out"=w434:errorcluster, "Image Out"=w438:T1)  [unwired: 8 in]
        n149 = local write "Camera"(w438) -> ()
      }
    }
  }
  n150 = Unregister For Events(event registration refnum=w11, error in=w9) -> (error out=w12:errorcluster)
  n151 = Merge Errors(w12, w15, w3) -> (w13:errorcluster)
  n152 = call "Destroy User Event - Stop.vi"("error in (no error)"=w13, "User Event - Stop"=w7) -> ("error out"=w10:errorcluster)  [unwired: 9 in]
  n153 = disable-structure shown="Default" {
    disable-tunnel: w10 -> [_ _]
    frame condition #0 (active) {
    }
    frame condition #1 {
      # "Call Quit LabVIEW if running as a built application."
      n154 = Quit LabVIEW() -> ()  [unwired: 1 in]
    }
  }
